vi "Read Variant.vi"(8 "error in (no error)":errorcluster, 11 "Message Data in":refnum<class "Message Data.lvclass">) -> (0 "error out":errorcluster, 2 "Variant":variant, 3 "Message Data out":refnum<class "Message Data.lvclass">)   [LabVIEW 2023, in "Message Data.lvclass"]
uses:
  Message Data.lvclass
  Message Data.lvclass/Message Data.ctl
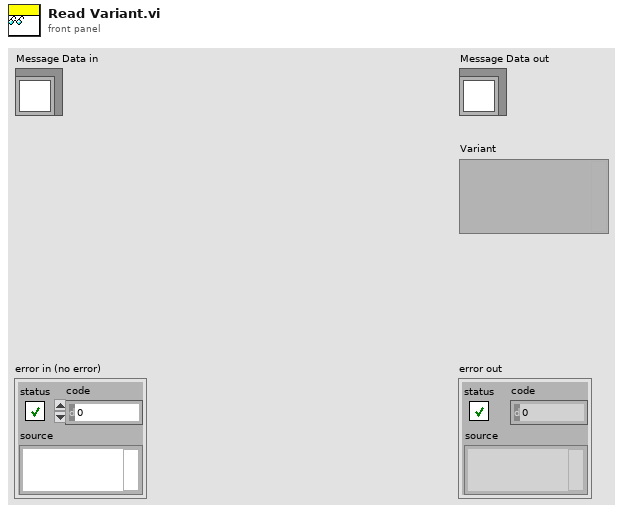
[diagram p1: front panel]
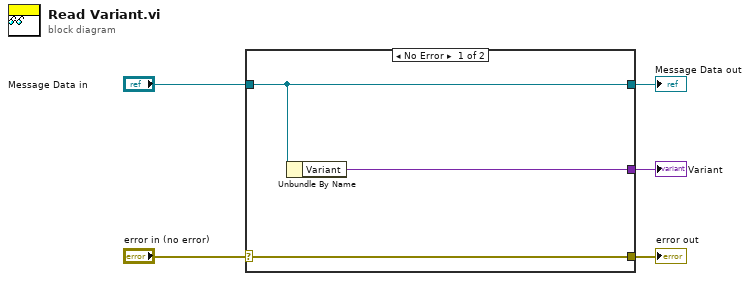
[diagram p0: block diagram]
diagram:
  n1 = case shown="No Error" "error in (no error)" {
    selector: "error in (no error)" -> [w8 w9]
    tunnel: [w8 w9] -> w4
    tunnel: [w7 w10] -> w2
    tunnel: "Message Data in" -> [w7 w10]
    tunnel: [w6 _] -> w1
    frame No Error {
      n2 = Unbundle By Name(w7) -> ("Variant"=w6:variant)
    }
    frame Error {
    }
  }
  "error out" <- w4
  "Message Data out" <- w2
  "Variant" <- w1
